vi "Load Hardware.vi"(8 "error in (no error)":errorcluster, 10 "Program only changes":bool=TRUE, 11 "DDS in":refnum<class "DDS.lvclass">) -> (0 "error out":errorcluster, 3 "DDS out":refnum<class "DDS.lvclass">)   [LabVIEW 2013, in "DDS.lvclass"]
uses:
  DDS.lvclass
  DDS.lvclass/DDS.ctl
  DDS9954_v2013.lvlib
panel:
  out "Program?":bool
  out "Names encountered":string[](array[string])
  out "Last HWI array":T1(array[cluster])
  out "FT_Status":u32(ring) items=["FT_OK", "FT_INVALID_HANDLE", "FT_DEVICE_NOT_FOUND", "FT_DEVICE_NOT_OPENED", "FT_IO_ERROR", "FT_INSUFFICIENT_RESOURCES", "FT_INVALID_PARAMETER", "FT_INVALID_BAUD_RATE", "FT_DEVICE_NOT_OPENED_FOR_ERASE", "FT_DEVICE_NOT_OPENED_FOR_WRITE", "FT_FAILED_TO_WRITE_DEVICE", "FT_EEPROM_READ_FAILED", "FT_EEPROM_WRITE_FAILED", "FT_EEPROM_ERASE_FAILED", "FT_EEPROM_NOT_PRESENT", "FT_EEPROM_NOT_PROGRAMMED", "FT_INVALID_ARGS", "FT_NOT_SUPPORTED", "FT_OTHER_ERROR"]
  in  "Leave DDS handles open?":bool
  out "Bytes Written":u32
  out "Characters to FPGA":string
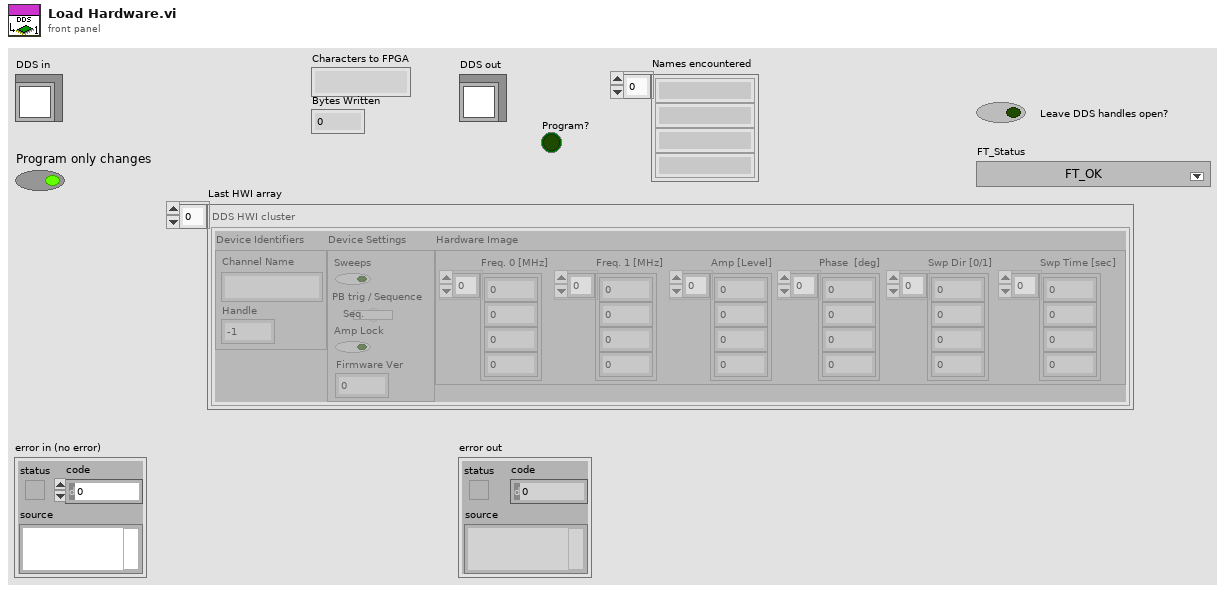
[diagram p1: front panel]
types:
  T1 = cluster{"Device Identifiers":cluster{"Channel Name":string, "Handle":i64}, "Device Settings":cluster{"Sweeps":bool, "PB trig / Sequence":bool, "Amp Lock":bool, "Firmware Ver":dbl}, "Hardware Image":cluster{"Freq. 0 [MHz]":dbl[], "Freq. 1 [MHz]":dbl[], "Amp [Level]":dbl[], "Phase  [deg]":dbl[], "Swp Dir [0/1]":i32[], "Swp Time [sec]":dbl[]}}[]
  T2 = cluster{"Sweeps":bool, "PB trig / Sequence":bool, "Amp Lock":bool, "Firmware Ver":dbl}
  T3 = cluster{"Freq. 0 [MHz]":dbl[], "Freq. 1 [MHz]":dbl[], "Amp [Level]":dbl[], "Phase  [deg]":dbl[], "Swp Dir [0/1]":i32[], "Swp Time [sec]":dbl[]}
  T4 = cluster{"Device Identifiers":cluster{"Channel Name":string, "Handle":i64}, "Device Settings":cluster{"Sweeps":bool, "PB trig / Sequence":bool, "Amp Lock":bool, "Firmware Ver":dbl}, "Hardware Image":cluster{"Freq. 0 [MHz]":dbl[], "Freq. 1 [MHz]":dbl[], "Amp [Level]":dbl[], "Phase  [deg]":dbl[], "Swp Dir [0/1]":i32[], "Swp Time [sec]":dbl[]}}
  T5 = cluster{"Freq. 0 [MHz]":dbl[], "Freq. 1 [MHz]":dbl[], "Amp [Level]":dbl[], "Phase  [deg]":dbl[], dbl[], "Swp Dir [0/1]":i32[], "Sweeps":bool, "Amp Lock":bool, bool, "Firmware Ver":dbl}
  T6 = cluster{"Device Description":string, "Handle In":i64}
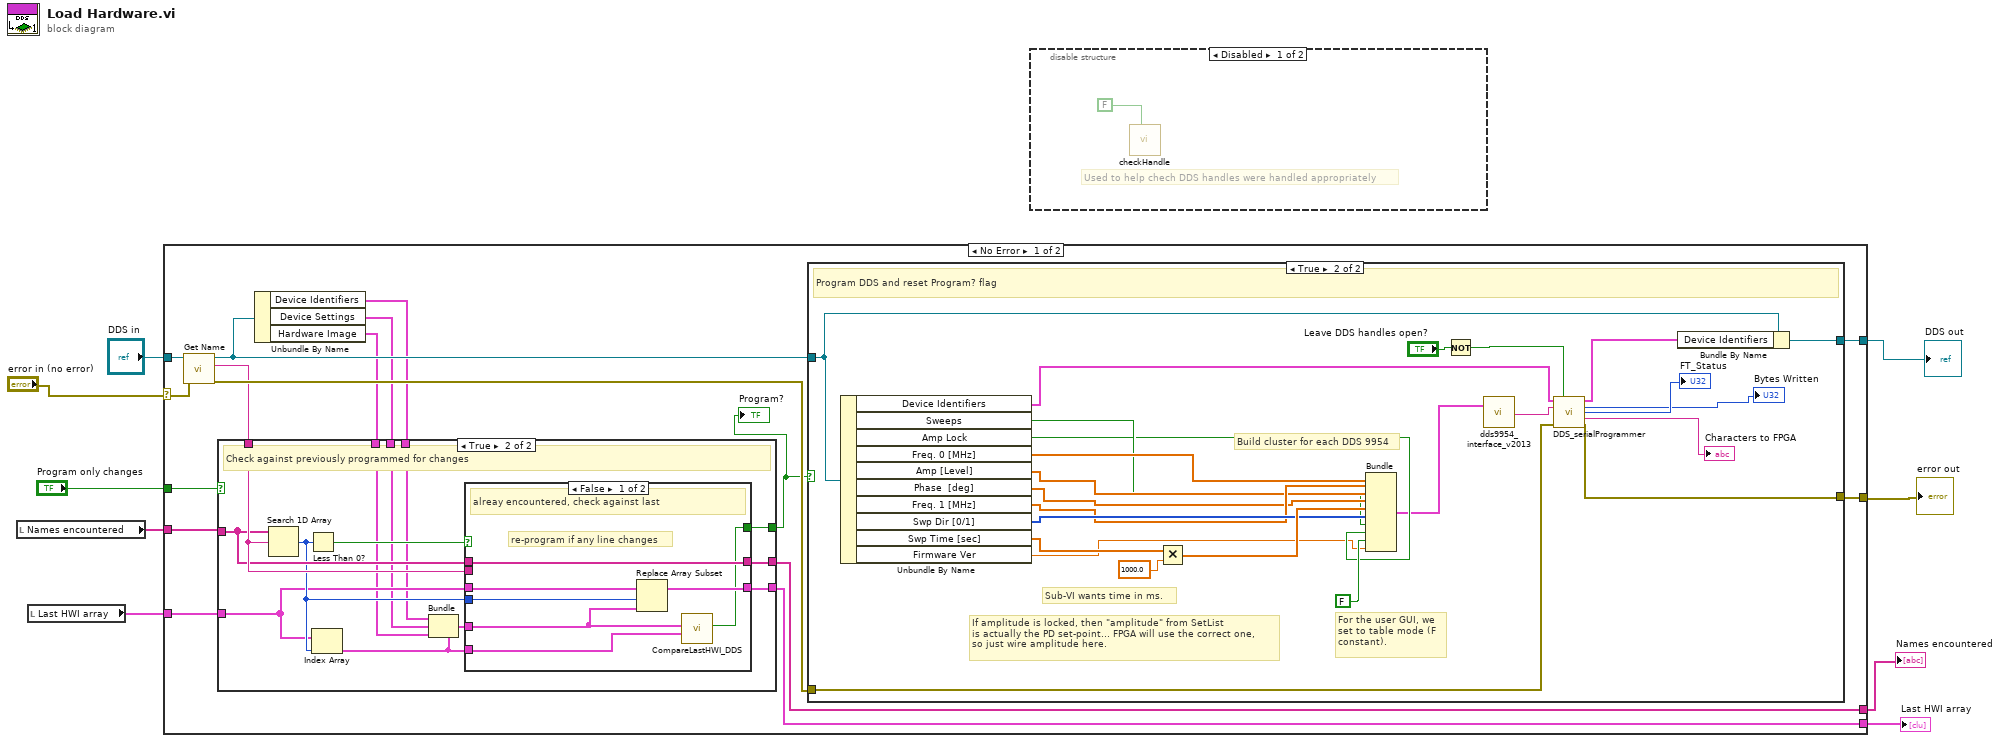
[diagram p0: block diagram]
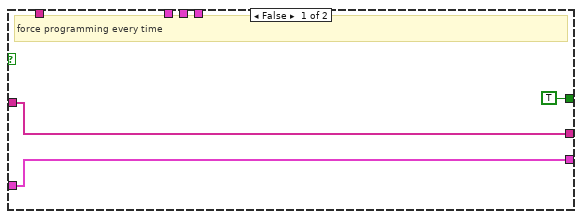
[diagram p3: hidden frame]
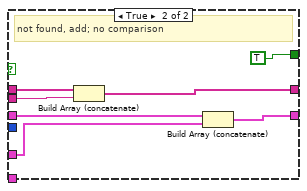
[diagram p4: hidden frame]
diagram:
  n1 = local read "Names encountered"() -> (w4:string[])
  n2 = local read "Last HWI array"() -> (w3:T1)
  n3 = case shown="No Error" "error in (no error)" {
    selector: "error in (no error)" -> [w21 w85]
    tunnel: [w25 w85] -> w8
    tunnel: [w24 w86] -> w6
    tunnel: "DDS in" -> [w23 w86]
    tunnel: "Program only changes" -> [w10 _]
    tunnel: w4 -> [w19 w83]
    tunnel: w3 -> [w18 w84]
    tunnel: [w13 w84] -> w1
    tunnel: [w12 w83] -> w2
    frame No Error {
      n4 = call-dynamic "Get Name.vi"("error in (no error)"=w21, "Device in"=w23) -> ("error out"=w22:errorcluster, "Name"=w20:string, "Device out"=w17:refnum<class "DDS.lvclass">)  [unwired: 7 in]
      n5 = Unbundle By Name(w17) -> ("Device Identifiers"=w16:cluster{"Channel Name":string, "Handle":i64}, "Device Settings"=w15:T2, "Hardware Image"=w14:T3)
      n6 = case shown="True" w10 {
        tunnel: [TRUE ("Diff?") w41] -> w11
        tunnel: [w28 w40] -> w12
        tunnel: w18 -> [w27 w34]
        tunnel: [w27 w39] -> w13
        tunnel: w16 -> [_ w32]
        tunnel: w20 -> [_ w37]
        tunnel: w19 -> [w28 w36]
        tunnel: w15 -> [_ w31]
        tunnel: w14 -> [_ w30]
        frame False {
          # "force programming every time"
        }
        frame True {
          # "Check against previously programmed for changes"
          n7 = Search 1D Array(1D array=w36, element=w37) -> (index of element=w35:i32)  [unwired: 1 in]
          n8 = Less Than 0?(x=w35) -> (x < 0?=w38:bool)
          n9 = Index Array(array=w34, index=w35) -> (element=w33:T4)
          n10 = Bundle(cluster=w33, "Device Identifiers"=w32, "Device Settings"=w31, "Hardware Image"=w30) -> (w29:T4)
          n11 = case shown="False" w38 {
            tunnel: w37 -> [_ w54]
            tunnel: w36 -> [w48 w55]
            tunnel: [w48 w53] -> w40
            tunnel: [w42 TRUE] -> w41
            tunnel: w34 -> [w47 w50]
            tunnel: w35 -> [w46 _]
            tunnel: [w45 w51] -> w39
            tunnel: w33 -> [w43 _]
            tunnel: w29 -> [w44 w49]
            frame False {
              # "re-program if any line changes"
              # "alreay encountered, check against last"
              n12 = Replace Array Subset(array=w47, new element=w44, index=w46) -> (w45:T1)
              n13 = call "CompareLastHWI_DDS.vi"("Last DDS HWI cluster"=w43, "DDS HWI cluster"=w44) -> ("change?"=w42:bool)  [unwired: 9 in]
            }
            frame True {
              # "not found, add; no comparison"
              n14 = Build Array (concatenate)(w55, w54) -> (w53:string[])
              n15 = Build Array (concatenate)(w50, w49) -> (w51:T1)
            }
          }
        }
      }
      "Program?" <- w11
      n16 = case shown="True" w11 {
        tunnel: w22 -> [w56 w65]
        tunnel: [w56 w58] -> w25
        tunnel: w17 -> [w57 w64]
        tunnel: [w57 w59] -> w24
        frame False {
          # "No need to program: (Program only changes = TRUE, and Program? = FALSE)"
        }
        frame True {
          # "Sub-VI wants time in ms."
          # "Build cluster for each DDS 9954"
          # "For the user GUI, we\nset to table mode (F \nconstant)."
          # "If amplitude is locked, then \"amplitude\" from SetList\nis actually the PD set-point... FPGA will use the correct one,\nso just wire amplitude here."
          # "Program DDS and reset Program? flag"
          n17 = Unbundle By Name(w64) -> ("Device Identifiers"=w68:cluster{"Channel Name":string, "Handle":i64}, "Sweeps"=w73:bool, "Amp Lock"=w72:bool, "Freq. 0 [MHz]"=w74:dbl[], "Amp [Level]"=w75:dbl[], "Phase  [deg]"=w76:dbl[], "Freq. 1 [MHz]"=w77:dbl[], "Swp Dir [0/1]"=w78:i32[], "Swp Time [sec]"=w79:dbl[], "Firmware Ver"=w67:dbl)
          n18 = Multiply(x=w79, y=1000.0) -> (x*y=w81:dbl[])
          n19 = Bundle("Freq. 0 [MHz]"=w74, "Freq. 1 [MHz]"=w77, "Amp [Level]"=w75, "Phase  [deg]"=w76, w81, "Swp Dir [0/1]"=w78, "Sweeps"=w73, "Amp Lock"=w72, FALSE, "Firmware Ver"=w67) -> (w66:T5)  [unwired: 1 in]
          n20 = Not(x="Leave DDS handles open?") -> (.not. x?=w69:bool)
          n21 = call "dds9954_interface_v2013.vi"("DDS9954 Interface"=w66) -> ("Characters to FPGA"=w62:string)  [unwired: 17 in, 1 out]
          n22 = call "DDS_serialProgrammer.vi"("Device In"=w68, "Reinitialize DDS"=w69, "Characters to FPGA"=w62, "error in"=w65) -> ("Device Out"=w63:T6, "Bytes Written"=→"Bytes Written":u32, "FT_Status"=→"FT_Status":u32, "Characters written to FPGA"=→"Characters to FPGA":string, "error out"=w58:errorcluster)  [unwired: 7 in]
          n23 = Bundle By Name(cluster=w64, "Device Identifiers"=w63) -> (w59:refnum<class "DDS.lvclass">)
        }
      }
    }
    frame Error {
    }
  }
  "error out" <- w8
  "DDS out" <- w6
  "Last HWI array" <- w1
  "Names encountered" <- w2
  n24 = disable-structure shown="Disabled" {
    frame Disabled {
      # "Used to help chech DDS handles were handled appropriately"
      n25 = call "checkHandle.vi"("Close all open DDS devices?"=FALSE) -> ()  [unwired: 9 in, 2 out]
    }
    frame Enabled {
    }
  }
